vi "Async Stream ReadDI Launcher.vi"(8 "error in (no error)":errorcluster, 11 "DIOSessions In":T1={"Array of DI Sessions"=[], "Array of DO Sessions"=[], "Stream ReadDI"={"gRPCid ReadDI"=0, "DISessionName"="", "Stream Status ReadDI"=FALSE, "Async Stop ReadDI Queue"=refnum, "DI Task"="", "ms to wait"=500}}) -> (0 "error out":errorcluster, 3 "DIOSessions Out":T1={"Array of DI Sessions"=[], "Array of DO Sessions"=[], "Stream ReadDI"={"gRPCid ReadDI"=0, "DISessionName"="", "Stream Status ReadDI"=FALSE, "Async Stop ReadDI Queue"=refnum, "DI Task"="", "ms to wait"=500}})   [LabVIEW 2019, in "ctet_dio_User Library.lvlib"]
uses:
  ctet_dio_User Library.lvlib
  Types/DIOSessions.ctl
  Types/DISession.ctl
  Types/DOSession.ctl
  Types/StreamReadDI.ctl
  Servers/ctet_dio/gRPC lvSupport/Server API/typeDefs/grpcId.ctl
  Servers/ctet_dio/gRPC lvSupport/gprc-lvsupport.lvlib
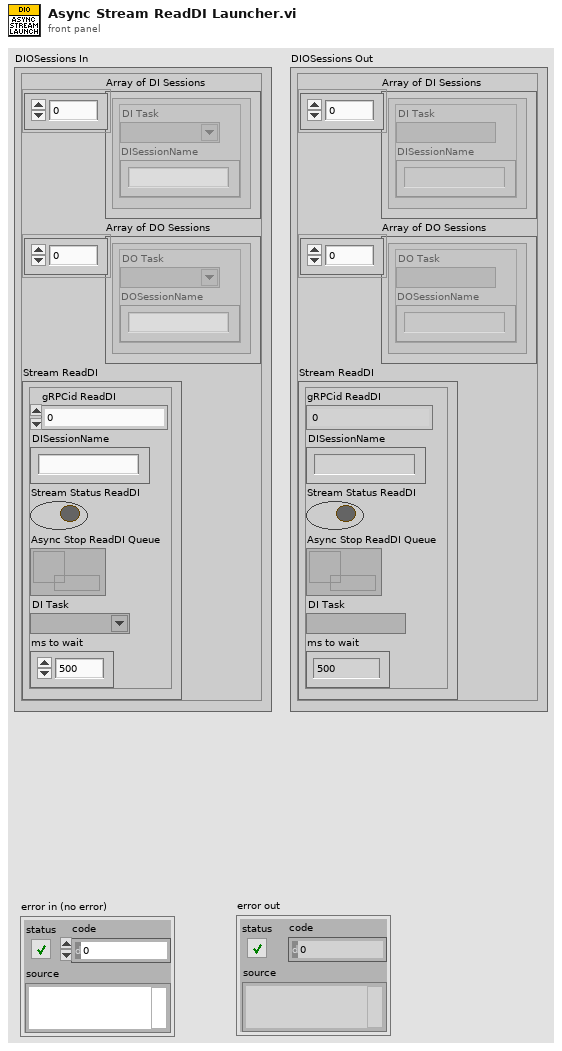
[diagram p1: front panel]
types:
  T1 = typedef "ctet_dio_User Library.lvlib/DIOSessions.ctl" = cluster{"Array of DI Sessions":T2[], "Array of DO Sessions":T3[], "Stream ReadDI":T4}
  T2 = typedef "ctet_dio_User Library.lvlib/DISession.ctl" = cluster{"DI Task":refnum<k21>, "DISessionName":string}
  T3 = typedef "ctet_dio_User Library.lvlib/DOSession.ctl" = cluster{"DO Task":refnum<k21>, "DOSessionName":string}
  T4 = typedef "ctet_dio_User Library.lvlib/StreamReadDI.ctl" = cluster{"gRPCid ReadDI":T5, "DISessionName":string, "Stream Status ReadDI":bool, "Async Stop ReadDI Queue":refnum<queue>, "DI Task":refnum<k21>, "ms to wait":u32}
  T5 = typedef "ctet_dio.lvlib/gprc-lvsupport.lvlib/grpcId.ctl" = u64
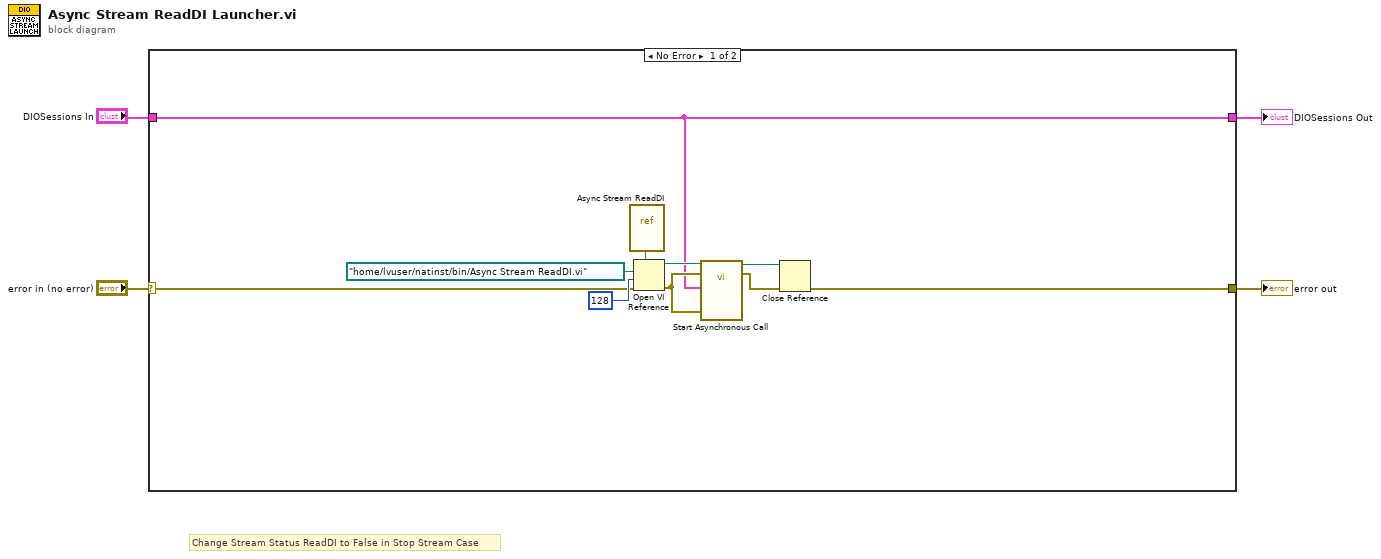
[diagram p0: block diagram]
diagram:
  # "Change Stream Status ReadDI to False in Stop Stream Case"
  n1 = case shown="No Error" "error in (no error)" {
    selector: "error in (no error)" -> [w6 w16]
    tunnel: [w7 w16] -> w4
    tunnel: "DIOSessions In" -> [w8 w15]
    tunnel: [w8 w15] -> w1
    frame No Error {
      n2 = vi-ref "Async Stream ReadDI.vi"() -> (w5:refnum<vi>)
      n3 = Open VI Reference(type specifier VI Refnum (for type only)=w5, vi path=path "/home/lvuser/natinst/bin/Async Stream ReadDI.vi", options=128, error in (no error)=w6) -> (vi reference=w14:refnum<vi>, error out=w9:errorcluster)  [unwired: 2 in]
      n4 = call-by-ref "Start Asynchronous Call"(reference=w14, error in=w9, 8:"error in (no error)"=w9, "DIOSessions In"=w8) -> (reference out=w13:refnum<vi>, error out=w12:errorcluster)  [unwired: 9 in, 1 out]
      n5 = Close Reference(reference=w13, error in (no error)=w12) -> (error out=w7:errorcluster)
    }
    frame Error {
    }
  }
  "error out" <- w4
  "DIOSessions Out" <- w1
